vi "error_check_probe_freq_sweep.vi"(10 "f in":T1, 11 "Boolean":bool) -> (3 "f out":T1)   [LabVIEW 2017]
uses:
  controls/State.ctl
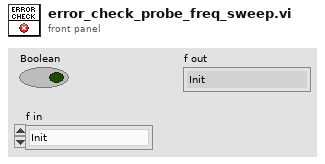
[diagram p1: front panel]
types:
  T1 = typedef "State.ctl" = enum16{"Init", "Idle", "Starting Meas", "Running", "Stopping Meas", "Shutting down"}
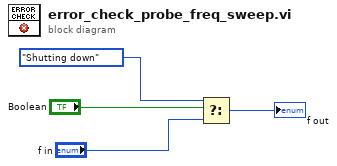
[diagram p0: block diagram]
diagram:
  n1 = Select(t=State."Shutting down", s="Boolean", f="f in") -> (s? t:f=→"f out":T1)
